vi "dfd_FXP PtByPt Direct FIR Transposed.vi"(6 "state in":i64[](array[numeric]), 7 "FXPOPs":T5[](array[typedef]) {"source" items=["Coef a/k"=0, "Coef b/v"=7, "Input"=1, "Output"=2, "Multiplicand"=3, "Product"=4, "Sum"=5, "Delay"=6, "Gain"=8]}, 8 "filtering statistics in":T3(array[cluster]) {"statistics information"."min value" format="%.2f"; "statistics information"."max value" format="%.2f"; "Quantizer Source" items=["Coefficients a/k"=0, "Coefficients b/v"=7, "Input"=1, "Output"=2, "Multiplicand"=3, "Product"=4, "Sum"=5, "Delay"=6]}, 10 "coef b":T4, 11 "x":T7={"value"=0, "wl"=0, "iwl"=0, "Signed"=TRUE} {"value" format="%.0x"}) -> (0 "filtering statistics out":T3(array[cluster]) {"statistics information"."min value" format="%.2f"; "statistics information"."max value" format="%.2f"; "Quantizer Source" items=["Coefficients a/k"=0, "Coefficients b/v"=7, "Input"=1, "Output"=2, "Multiplicand"=3, "Product"=4, "Sum"=5, "Delay"=6]}, 3 "filtered x":T7={"value"=0, "wl"=0, "iwl"=0, "Signed"=TRUE} {"value" format="%.0x"}, 4 "state out":i64[](array[numeric]))   [LabVIEW 2017, in "NI_DigFilter_FXP.lvlib"]
uses:
  <vilib>/addons/Digital Filter Design/NI_DigFilter_FXP.lvlib
  <vilib>/addons/Digital Filter Design/_Objects.llb/dfd_DFXP Data Type (scaler).ctl
  <vilib>/addons/Digital Filter Design/_Objects.llb/dfd_DFXP Operation Parameter.ctl
  <vilib>/addons/Digital Filter Design/_Objects.llb/dfd_Internal Quantization Srcs.ctl
  <vilib>/addons/Digital Filter Design/_Objects.llb/dfd_DFXP Data Type (vector).ctl
  <vilib>/addons/Digital Filter Design/_Objects.llb/DFD Quantization Sources.ctl
  <vilib>/addons/Digital Filter Design/_Objects.llb/DFD FXP Statistics Data.ctl
  <vilib>/addons/Digital Filter Design/NI_DigFilterLicensed.lvlib
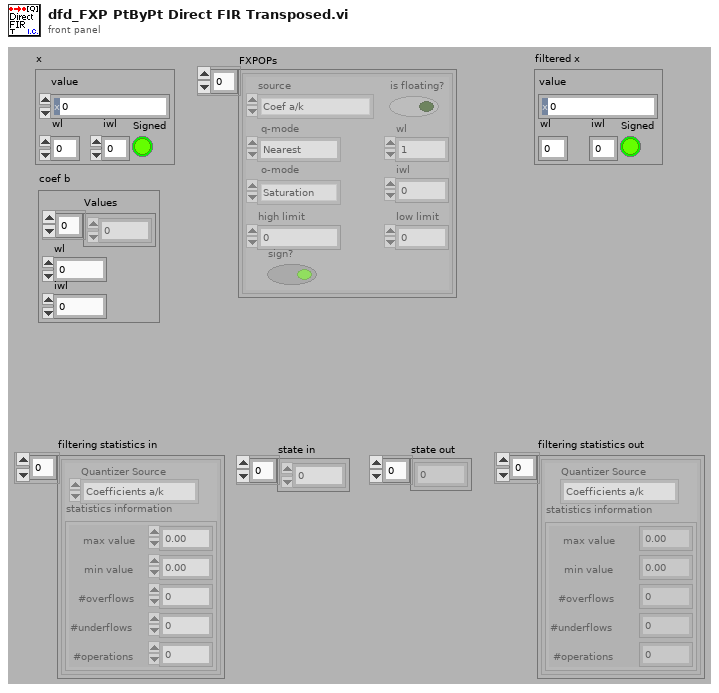
[diagram p1: front panel]
types:
  T1 = typedef "NI_DigFilterLicensed.lvlib/DFD Quantization Sources.ctl" = u16
  T2 = typedef "NI_DigFilterLicensed.lvlib/DFD FXP Statistics Data.ctl" = cluster{"max value":ext, "min value":ext, "#overflows":i32, "#underflows":i32, "#operations":i32}
  T3 = cluster{"Quantizer Source":T1, "statistics information":T2}[]
  T4 = typedef "dfd_DFXP Data Type (vector).ctl" = cluster{"Values":i64[], "wl":i16, "iwl":i16}
  T5 = typedef "dfd_DFXP Operation Parameter.ctl" = cluster{"source":T6, "is floating?":bool, "o-mode":enum16{"Saturation", "Wrap"}, "q-mode":enum16{"Nearest", "Truncation"}, "wl":i16, "high limit":i64, "low limit":i64, "iwl":i16, "sign?":bool}
  T6 = typedef "NI_DigFilterLicensed.lvlib/dfd_Internal Quantization Srcs.ctl" = u16
  T7 = typedef "dfd_DFXP Data Type (scaler).ctl" = cluster{"value":i64, "wl":i16, "iwl":i16, "Signed":bool}
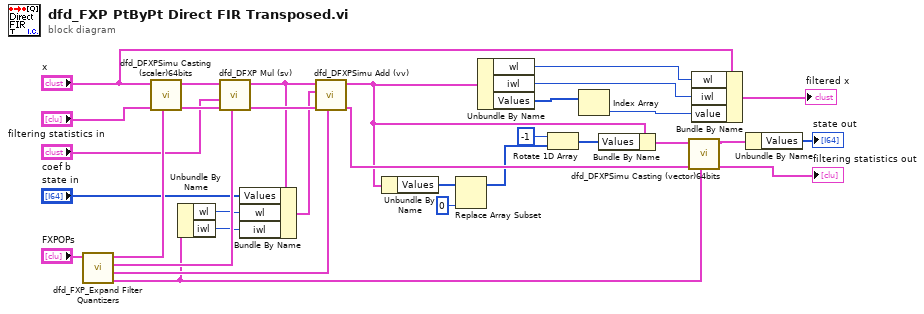
[diagram p0: block diagram]
diagram:
  n1 = call <vilib>:"dfd_FXP_Expand Filter Quantizers.vi"("FXPOPs"="FXPOPs") -> ("Delay"=w7:T5, "Sum"=w25:T5, "Product"=w26:T5, "Multiplicand"=w27:T5)  [unwired: 7 out]
  n2 = call <vilib>:"dfd_DFXPSimu Casting (scaler)64bits.vi"("op params"=w27, "filtering statistics in"="filtering statistics in", "Value in"="x") -> ("filtering statistics out"=w29:T3, "Value out"=w22:T7)  [unwired: 2 in, 5 out]
  n3 = Unbundle By Name(w7) -> ("wl"=w6:i16, "iwl"=w5:i16)
  n4 = call <vilib>:"dfd_DFXP Mul (sv).vi"("op params"=w26, "filtering statistics in"=w29, "Value in 2"="coef b", "Value in"=w22) -> ("filtering statistics out"=w24:T3, "Value out"=w8:T4)  [unwired: 2 in, 4 out]
  n5 = Bundle By Name(cluster=w8, "Values"="state in", "wl"=w6, "iwl"=w5) -> (w9:T4)
  n6 = call <vilib>:"dfd_DFXPSimu Add (vv).vi"("op params"=w25, "filtering statistics in"=w24, "values in 2"=w9, "values in 1"=w8) -> ("filtering statistics out"=w23:T3, "values out"=w18:T4)  [unwired: 6 out]
  n7 = Unbundle By Name(w18) -> ("Values"=w2:i64[])
  n8 = Replace Array Subset(array=w2, new element=i64 0 ("new element/subarray")) -> (w1:i64[])  [unwired: 1 in]
  n9 = Unbundle By Name(w18) -> ("wl"=w13:i16, "iwl"=w12:i16, "Values"=w17:i64[])
  n10 = Rotate 1D Array(1:w1, 2:-1 ("n")) -> (0:w21:i64[])
  n11 = Index Array(array=w17) -> (element=w16:i64)  [unwired: 1 in]
  n12 = Bundle By Name(cluster=w18, "Values"=w21) -> (w20:T4)
  n13 = call <vilib>:"dfd_DFXPSimu Casting (vector)64bits.vi"("op params"=w7, "filtering statistics in"=w23, "Value in"=w20) -> ("filtering statistics out"=→"filtering statistics out":T3, "Value out"=w11:T4)  [unwired: 1 in, 6 out]
  n14 = Bundle By Name(cluster="x", "wl"=w13, "iwl"=w12, "value"=w16) -> (→"filtered x":T7)
  n15 = Unbundle By Name(w11) -> ("Values"=→"state out":i64[])
